vi "Get Transaction by Row.vi"(8 "error in (no error)":errorcluster, 10 "Row":u32, 11 "Statement in":refnum<class "TransactionList.lvclass">) -> (0 "error out":errorcluster, 2 "Transaction.lvclass":refnum<class "Transaction.lvclass">, 3 "Statement out":refnum<class "TransactionList.lvclass">)   [LabVIEW 2018, in "TransactionList.lvclass"]
uses:
  TransactionList.lvclass
  Transaction/Transaction.lvclass
  TransactionList.lvclass/TransactionList.ctl
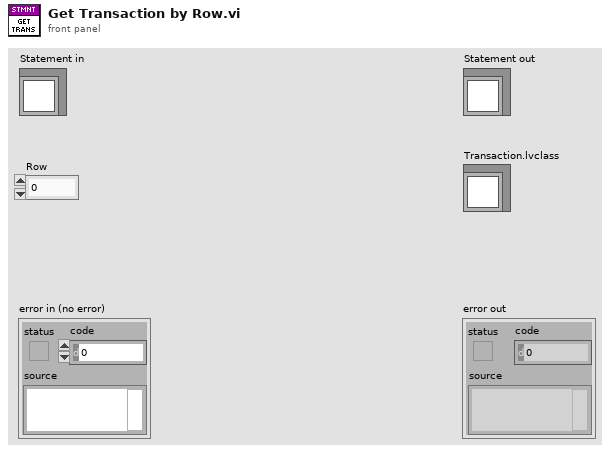
[diagram p1: front panel]
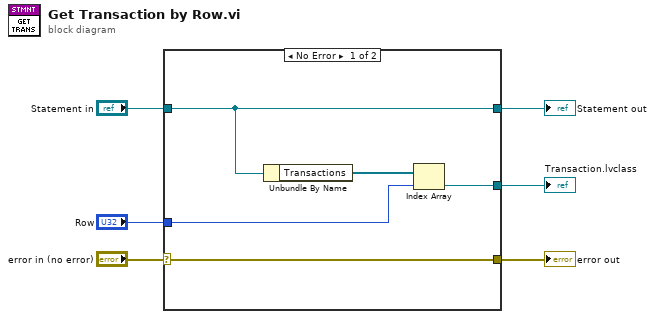
[diagram p0: block diagram]
diagram:
  n1 = case shown="No Error" "error in (no error)" {
    selector: "error in (no error)" -> [w11 w13]
    tunnel: [w11 w13] -> w5
    tunnel: [w10 w12] -> w3
    tunnel: "Statement in" -> [w10 w12]
    tunnel: "Row" -> [w8 _]
    tunnel: [w7 _] -> w1
    frame No Error {
      n2 = Unbundle By Name(w10) -> ("Transactions"=w9:refnum<class "Transaction.lvclass">[])
      n3 = Index Array(array=w9, index=w8) -> (element=w7:refnum<class "Transaction.lvclass">)
    }
    frame Error {
    }
  }
  "error out" <- w5
  "Statement out" <- w3
  "Transaction.lvclass" <- w1
